vi "Tool Q LEIN controller relay task.vi"(0 "Controller addres":u8=42, 5 "current limit(0.2A)":dbl, 7 "outpuyt channel":u8, 9 "time (50 ms)":u16=50, 11 "error in (no error)":errorcluster) -> (4 "LEIN custom reply Q":T1, 15 "error out":errorcluster)   [LabVIEW 2011]
uses:
  LEINmaster/Defenitions/LEIN custom reply Q.ctl
  LEINmaster/Defenitions/LEIN Reply Holder.ctl
  LEINmaster/Defenitions/LEIN CMD Cluster.ctl
  LEINmaster/Defenitions/LEIN CMD List.ctl
  LEINmaster/Defenitions/LEIN Structure variations.ctl
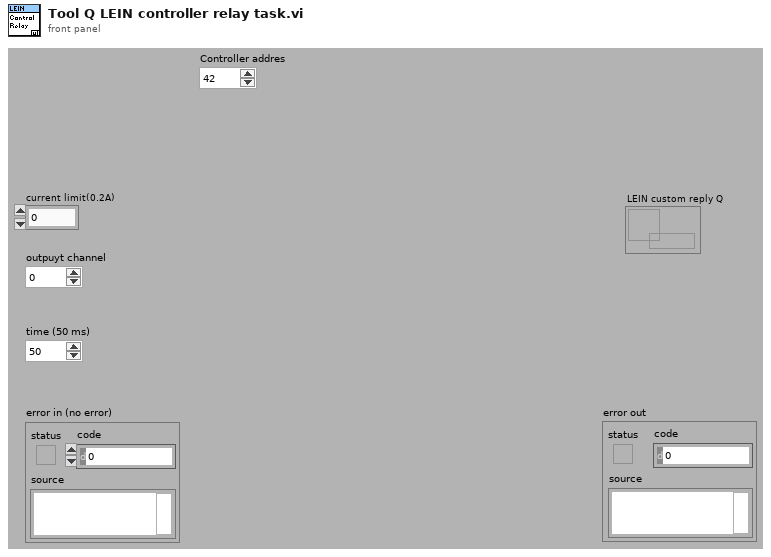
[diagram p1: front panel]
types:
  T1 = typedef "LEIN custom reply Q.ctl" = refnum<queue>
  T2 = typedef "LEIN Structure variations.ctl" = enum16{"LEIN08", "LEIN31", "LEIN63"}
  T3 = enum16{"big-endian, network order", "native, host order", "little-endian"}
  T4 = typedef "LEIN CMD Cluster.ctl" = cluster{"SID":u8, "ANF":bool, "CMD":T5, "DATA":u8[]}
  T5 = typedef "LEIN CMD List.ctl" = enum8{"ACTI", "TASK", "RES0", "STAT", "RES1", "RES2", "RES3", "USER"}
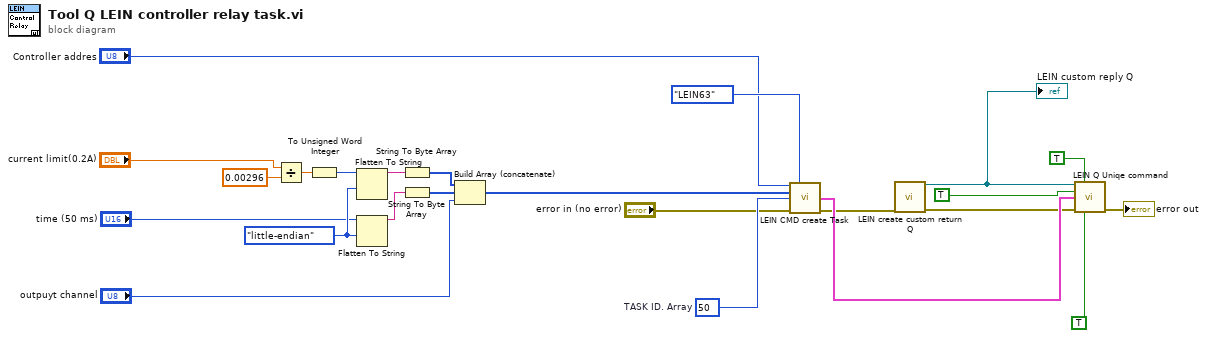
[diagram p0: block diagram]
diagram:
  w12 = u8 50  # TASK ID. Array
  w18 = T3."little-endian" ("byte order (0:big-endian, network order)")
  n1 = Divide(x="current limit(0.2A)", y=0.00296 ("x")) -> (x/y=w23:dbl)
  n2 = To Unsigned Word Integer(number=w23) -> (unsigned 16bit integer=w21:u16)
  n3 = Flatten To String(anything=w21, byte order (0:big-endian, network order)=w18) -> (data string=w20:string)  [unwired: 2 in, 2 out]
  n4 = Flatten To String(anything="time (50 ms)", byte order (0:big-endian, network order)=w18) -> (data string=w16:string)  [unwired: 2 in, 2 out]
  n5 = String To Byte Array(string=w20) -> (unsigned byte array=w19:u8[])
  n6 = String To Byte Array(string=w16) -> (unsigned byte array=w15:u8[])
  n7 = Build Array (concatenate)(w19, w15, "outpuyt channel") -> (w10:u8[])
  n8 = call "LEIN CMD create Task.vi"("SID"="Controller addres", "LEIN Variation"=LEIN_Structure_variations."LEIN63", "Data"=w10, "TASK ID"=w12, "error in (no error)"="error in (no error)") -> ("CMD"=w6:T4, "error out"=w5:errorcluster)  [unwired: 9 in]
  n9 = call "LEIN create custom return Q.vi"("error in (no error)"=w5) -> ("LEIN custom reply Q"=w3:T1, "error out"=w4:errorcluster)  [unwired: 13 in]
  "LEIN custom reply Q" <- w3
  n10 = call "LEIN Q Uniqe command.vi"("LEIN custom reply Q"=w3, "Retry on err (F)"=TRUE, "Custom Q(F)"=TRUE, "CMD"=w6, "error in"=w4, "priority(F)"=TRUE) -> ("error out"=→"error out":errorcluster)  [unwired: 9 in]
